vi "Voronoi_Boundary Edges Main.vi"(6 "Range":dbl[](array[numeric]), 8 "Center":dbl[](array[numeric]), 9 "P 3":dbl[](array[numeric]), 10 "P 2":dbl[](array[numeric]), 11 "P 1":dbl[](array[numeric])) -> (2 "End":dbl[](array[numeric]), 3 "Start":dbl[](array[numeric]))   [LabVIEW 2017, in "NI_AAL_Geometry.lvlib"]
uses:
  <vilib>/Analysis/NI_AAL_Geometry.lvlib
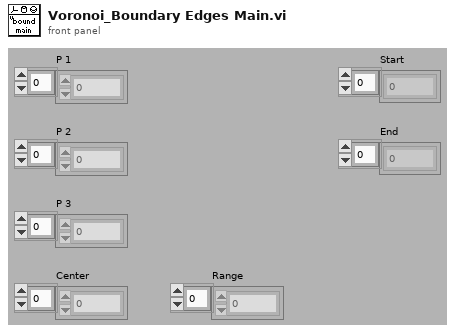
[diagram p1: front panel]
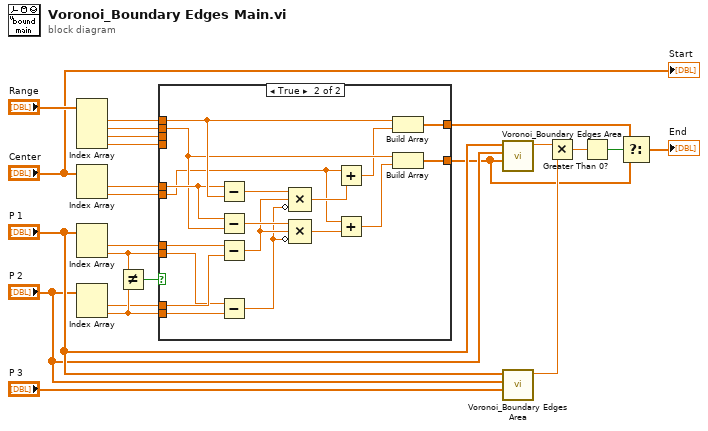
[diagram p0: block diagram]
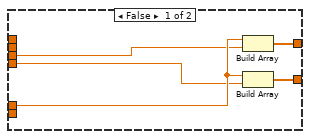
[diagram p2: hidden frame]
diagram:
  n1 = Index Array(array="Range") -> (element #1=w18:dbl, element #2=w17:dbl, element #3=w16:dbl, element #4=w15:dbl)  [unwired: 4 in]
  n2 = Index Array(array="Center") -> (element #1=w21:dbl, element #2=w13:dbl)  [unwired: 2 in]
  n3 = Index Array(array="P 1") -> (element #1=w12:dbl, element #2=w20:dbl)  [unwired: 2 in]
  n4 = Index Array(array="P 2") -> (element #1=w11:dbl, element #2=w19:dbl)  [unwired: 2 in]
  n5 = Not Equal?(x=w20, y=w19) -> (x != y?=w23:bool)
  n6 = case shown="True" w23 {
    tunnel: w21 -> [w26 w41]
    tunnel: w12 -> [_ w46]
    tunnel: w20 -> [_ w43]
    tunnel: w11 -> [_ w45]
    tunnel: w19 -> [_ w44]
    tunnel: w18 -> [_ w42]
    tunnel: w17 -> [_ w36]
    tunnel: w16 -> [w25 _]
    tunnel: w15 -> [w24 _]
    tunnel: [w28 w35] -> w2
    tunnel: [w27 w34] -> w3
    tunnel: w13 -> [_ w31]
    frame False {
      n7 = Build Array(w26, w25) -> (w28:dbl[])
      n8 = Build Array(w26, w24) -> (w27:dbl[])
    }
    frame True {
      n9 = Subtract(x=w41, y=w42) -> (x-y=w40:dbl)
      n10 = Subtract(x=w41, y=w36) -> (x-y=w39:dbl)
      n11 = Subtract(x=w46, y=w45) -> (x-y=w38:dbl)
      n12 = Subtract(x=w43, y=w44) -> (x-y=w37:dbl)
      n13 = Compound Arithmetic op=MULTIPLY(w40, w38, invert w37) -> (w33:dbl)
      n14 = Compound Arithmetic op=MULTIPLY(w39, w38, invert w37) -> (w30:dbl)
      n15 = Add(x=w31, y=w33) -> (x+y=w32:dbl)
      n16 = Add(x=w31, y=w30) -> (x+y=w29:dbl)
      n17 = Build Array(w42, w32) -> (w35:dbl[])
      n18 = Build Array(w36, w29) -> (w34:dbl[])
    }
  }
  n19 = call <vilib>:"Voronoi_Boundary Edges Area.vi"("P 3"=w3, "P 2"="P 2", "P 1"="P 1") -> ("area"=w7:dbl)  [unwired: 8 out]
  n20 = call <vilib>:"Voronoi_Boundary Edges Area.vi"("P 3"="P 3", "P 2"="P 2", "P 1"="P 1") -> ("area"=w6:dbl)  [unwired: 8 out]
  n21 = Multiply(x=w7, y=w6) -> (x*y=w5:dbl)
  n22 = Greater Than 0?(x=w5) -> (x > 0?=w4:bool)
  n23 = Select(t=w2, s=w4, f=w3) -> (s? t:f=→"End":dbl[])
  "Start" <- "Center"
